vi "Motic Set RGB Offset.vi"(0 "camera":i32, 5 "r":i32, 7 "g":i32, 9 "b":i32, 11 "error in (no error)":errorcluster) -> (4 "camera out":i32, 15 "error out":errorcluster)   [LabVIEW 2012, in "MoticApi.lvlib"]
doc: "MOTICAPI bool Motic_SetRGBOffset(MUCam_Handle camera, int r, int g, int b);"
uses:
  MoticApi.lvlib
  MoticApi.dll
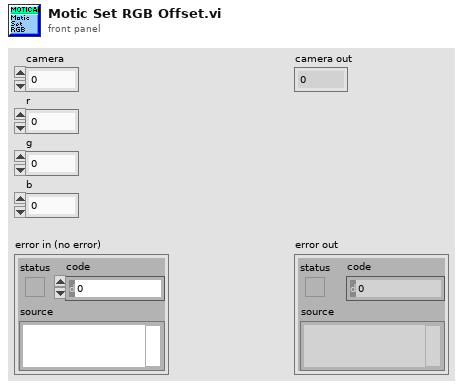
[diagram p1: front panel]
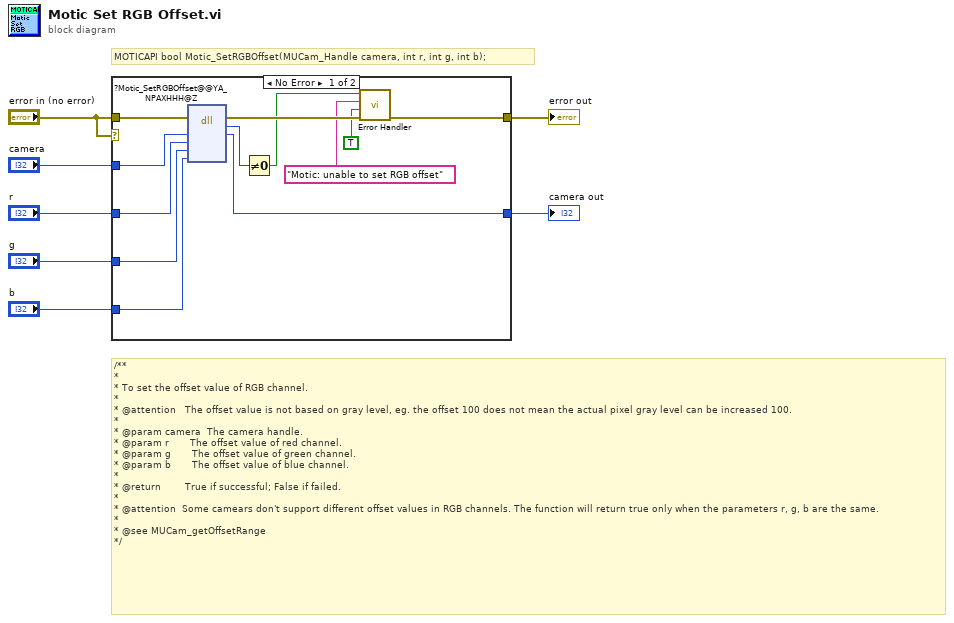
[diagram p0: block diagram]
diagram:
  # "/**\n*\n* To set the offset value of RGB channel.\n*\n* @attention   The offset value is not based on gray level, eg. the offset 100 does not mean the actual pixel gray level can be increased 100.\n*\n* @param camera  The camera handle.\n* @param r       The offset value of red channel.\n* @param g       The offset value of green channel.\n* @param b       The offset value of blue channel.\n*\n* @return        True if successful; False if failed.\n*\n* @attention  Some camears don't support different offset values in RGB channels. The function will return true only when the parameters r, g, b are the same.\n*\n* @see MUCam_getOffsetRange\n*/"
  # "MOTICAPI bool Motic_SetRGBOffset(MUCam_Handle camera, int r, int g, int b);"
  n1 = case shown="No Error" "error in (no error)" {
    tunnel: "camera" -> [w18 w20]
    tunnel: [w17 w20] -> w6
    tunnel: "r" -> [w16 _]
    tunnel: "g" -> [w15 _]
    tunnel: "b" -> [w14 _]
    tunnel: "error in (no error)" -> [w13 w21]
    tunnel: [w12 w21] -> w2
    frame No Error {
      n2 = dll-call lib="C:/Users/TTS-Digital/Desktop/MoticApi/MoticApi_git/MoticApi/MoticApi.*" fn="?Motic_SetRGBOffset@@YA_NPAXHHH@Z"(error in=w13, "camera"=w18, "r"=w16, "g"=w15, "b"=w14) -> (error out=w11:errorcluster, w19:u8, "camera"=w17:i32)  [unwired: 5 in, 1 out]
      n3 = Not Equal To 0?(x=w19) -> (x != 0?=w10:bool)
      n4 = call "Error Handler.vi"("error in (no error)"=w11, "Is warning?"=TRUE, "Error message"="Motic: unable to set RGB offset", "Function return"=w10) -> ("error out"=w12:errorcluster)  [unwired: 7 in]
    }
    frame Error {
    }
  }
  "camera out" <- w6
  "error out" <- w2
